vi "DSF.Engine.Timing.Iteration.Set.vi"(8 "error in (no error)":errorcluster, 10 "iteration":u64=1, 11 "Timing in":refnum<class "DSF.Engine.Timing.lvclass">) -> (0 "error out":errorcluster, 3 "Timing out":refnum<class "DSF.Engine.Timing.lvclass">)   [LabVIEW 2017, in "Data Sharing Framework Engine.lvlib" / "DSF.Engine.Timing.lvclass"]
uses:
  DSF.Engine.Timing.lvclass
  DSF.Engine.Timing.lvclass/DSF.Engine.Timing.ctl
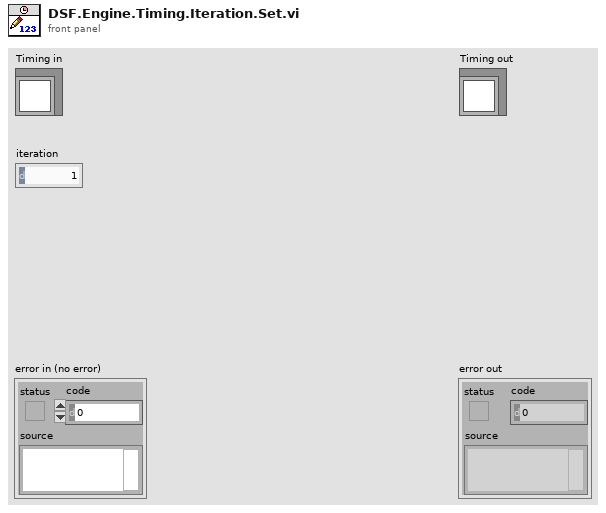
[diagram p1: front panel]
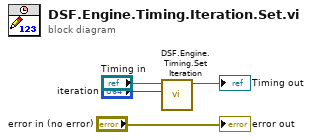
[diagram p0: block diagram]
diagram:
  n1 = call "DSF.Engine.Timing.Set Iteration.vi"("Iteration"="iteration", "Timing in"="Timing in") -> ("Timing out"=→"Timing out":refnum<class "DSF.Engine.Timing.lvclass">)  [unwired: 9 in]
  "error out" <- "error in (no error)"
